vi "BELKIN EAGLE RT Main V1.vi"() -> ()   [LabVIEW 2015]
uses:
  Stream/Controls/RT Status Refs.ctl
  <vilib>/userdefined/High Color/IMAQdx.ctl
  Stream/Controls/RT Streamer Queue element.ctl
  Stream/Controls/RT Streamer State.ctl
  Stream/LP Globals.vi
panel:
  out "Timings":u32[](array[numeric])
  in  "CamSession":T1="cam0"
  in  "AutoBalance":bool
  in  "SetParams":bool
  in  "StatusRefs":T2
  out "output cluster":T3
  in  "AlgoRate":u8=10
  out "FrameRate":dbl
  out "Image Dst Out":T4(plugin-control)
  out "MaxY":u32
  out "MaxX":u32
  out "MaxB":u32
  out "MaxA":u32
  out "HorCenter":u16
  out "VerCenter":u32
  out "Algo Time":u32
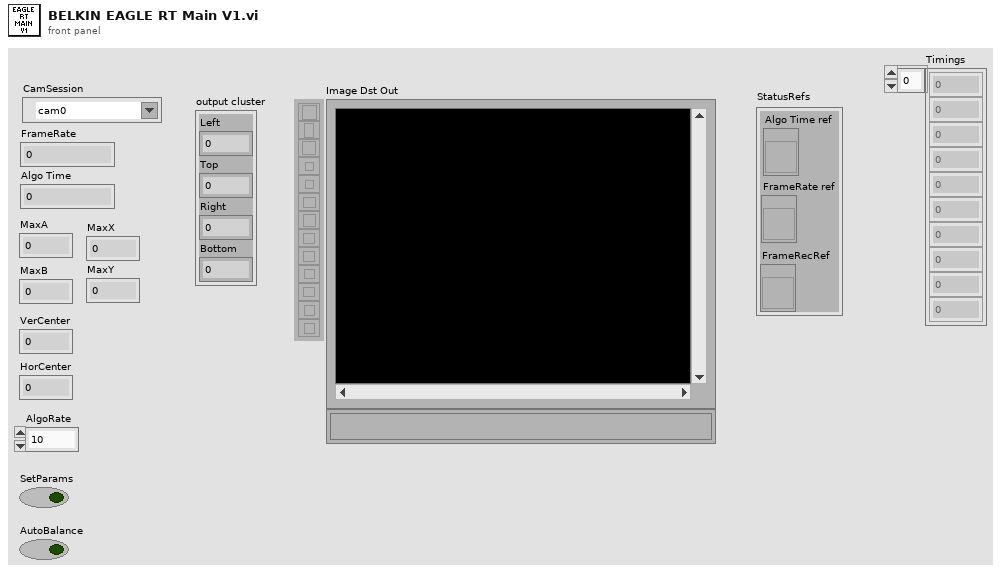
[diagram p1: front panel]
types:
  T1 = typedef "IMAQdx.ctl" = refnum<k21>
  T2 = typedef "RT Status Refs.ctl" = cluster{"Algo Time ref":refnum<vi>, "FrameRate ref":refnum<vi>, "FrameRecRef":refnum<vi>}
  T3 = cluster{"Left":i32, "Top":i32, "Right":i32, "Bottom":i32}
  T4 = typedef "IMAQ Image.ctl" = refnum<image>
  T5 = typedef "RT Streamer Queue element.ctl" = cluster{"CMD":T6, "Data":variant}
  T6 = typedef "RT Streamer State.ctl" = enum16{"Init", "Idle", "Stream", "Listen", "SetRefrashRate", "SendCmdAck", "SendCmdDone", "SendSysState", "StartRecord", "Error"}
  T7 = typedef "Image Type" = u32
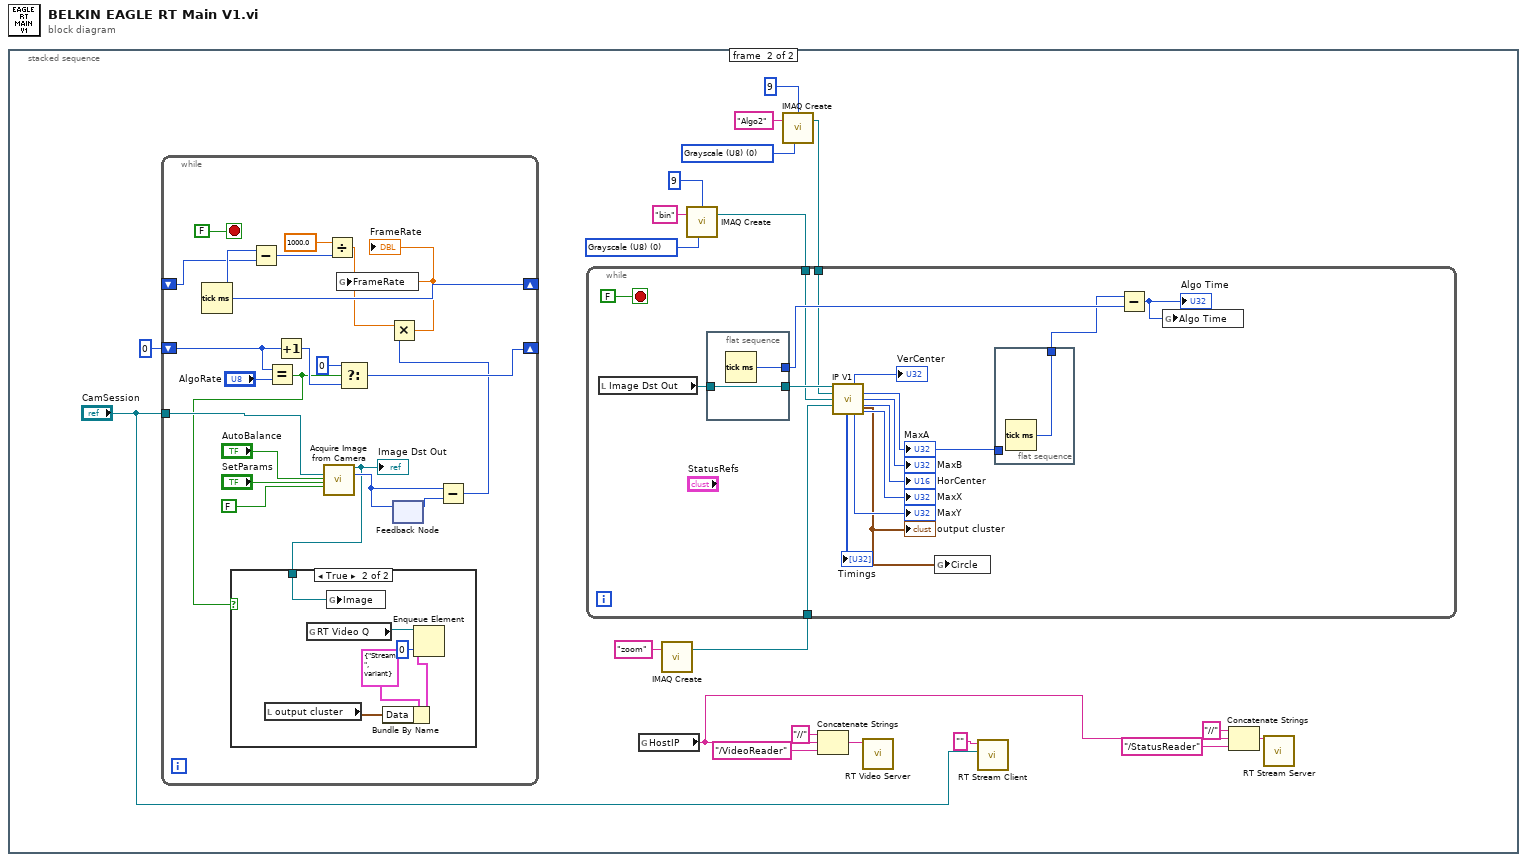
[diagram p0: block diagram]
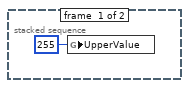
[diagram p2: hidden frame]
diagram:
  n1 = stacked-sequence {
    frame #0 {
      n2 = global write "LP Globals.vi" "UpperValue"(255 ("UpperValue")) -> ()
    }
    frame #1 {
      w8 = T7 0 items=["Grayscale (U8)", "Grayscale (I16)", "Grayscale (SGL)", "Complex (CSG)", "RGB (U32)", "HSL (U32)", "RGB (U64)", "Grayscale (U16)"] ("Image Type")
      w12 = T7 0 items=["Grayscale (U8)", "Grayscale (I16)", "Grayscale (SGL)", "Complex (CSG)", "RGB (U32)", "HSL (U32)", "RGB (U64)", "Grayscale (U16)"] ("Image Type")
      n3 = while {
        shift-right: [w60] -> _
        shift-left: _ -> [w59]
        shift-right: [w55] -> _
        shift-left: u8 0 -> [w57]
        tunnel: "CamSession" -> [w44]
        stop <- FALSE stop-if-true
        n4 = Tick Count (ms)() -> (millisecond timer value=w60:u32)
        n5 = Subtract(x=w60, y=w59) -> (x-y=w58:u32)
        n6 = Equal?(x=w57, y="AlgoRate") -> (x = y?=w43:bool)
        n7 = Increment(x=w57) -> (x+1=w56:u8)
        n8 = call "Acquire Image from Camera.vi"("Session In"=w44, "AutoBalance"="AutoBalance", "Set"="SetParams", "Stop (F)"=FALSE) -> ("Image Out"=w42:T4, "Buffer Number Out"=w48:u32)  [unwired: 20 in, 2 out]
        "Image Dst Out" <- w42
        n9 = case shown="True" w43 {
          tunnel: w42 -> [_ w64]
          frame False {
          }
          frame True {
            n10 = local read "output cluster"() -> (w65:T3)
            n11 = global read "LP Globals.vi" "RT Video Q"() -> (w68:refnum<queue>)
            n12 = global write "LP Globals.vi" "Image"(w64) -> ()
            n13 = Bundle By Name(cluster=T5 {"CMD"=enum."Stream", "Data"=variant} ("element"), "Data"=w65) -> (w66:T5)
            n14 = Enqueue Element(queue=w68, element=w66, timeout in ms (-1)=0) -> ()  [unwired: 1 in, 3 out]
          }
        }
        n15 = Divide(x=1000.0, y=w58) -> (x/y=w49:dbl)
        n16 = Select(t=u8 0, s=w43, f=w56) -> (s? t:f=w55:u8)
        n17 = feedback-in #1(w48) -> ()
        n18 = feedback #1() -> (w47:u32)  [unwired: 1 in]
        n19 = Subtract(x=w48, y=w47) -> (x-y=w46:u32)
        n20 = Multiply(x=w49, y=w46) -> (x*y=w45:dbl)
        "FrameRate" <- w45
        n21 = global write "LP Globals.vi" "FrameRate"(w45) -> ()
      }
      n22 = global read "LP Globals.vi" "HostIP"() -> (w13:string)
      n23 = call "IMAQ Create"("Image Name"="zoom") -> ("New Image"=w3:T4)  [unwired: 3 in, 2 out]
      n24 = call "IMAQ Create"("Border Size"=9, "Image Name"="bin", "Image Type"=w8) -> ("New Image"=w7:T4)  [unwired: 2 in, 1 out]
      n25 = call "IMAQ Create"("Border Size"=9, "Image Name"="Algo2", "Image Type"=w12) -> ("New Image"=w10:T4)  [unwired: 2 in, 1 out]
      n26 = while {
        tunnel: w10 -> [w29]
        tunnel: w7 -> [w28]
        tunnel: w3 -> [w25]
        stop <- FALSE stop-if-true
        n27 = local read "Image Dst Out"() -> (w23:T4)
        n28 = flat-sequence {
          tunnel: [w41] -> w32
          tunnel: w23 -> [w40]
          tunnel: [w40] -> w30
          frame #0 {
            n29 = Tick Count (ms)() -> (millisecond timer value=w41:u32)
          }
        }
        n30 = call "IP V1.vi"("Image In"=w30, "Image Dst"=w29, "BinImage"=w28, "Zoom Image"=w25) -> ("VerCenter"=→"VerCenter":u32, "MaxA"=w27:u32, "MaxB"=→"MaxB":u32, "HorCenter"=→"HorCenter":u16, "Timings"=→"Timings":u32[], "output cluster"=w22:T3, "MaxY"=→"MaxY":u32, "MaxX"=→"MaxX":u32)  [unwired: 1 in, 3 out]
        "MaxA" <- w27
        "output cluster" <- w22
        n31 = global write "LP Globals.vi" "Circle"(w22) -> ()
        n32 = flat-sequence {
          tunnel: [w39] -> w31
          tunnel: w27 -> [_]
          frame #0 {
            n33 = Tick Count (ms)() -> (millisecond timer value=w39:u32)
          }
        }
        n34 = Subtract(x=w31, y=w32) -> (x-y=w26:u32)
        "Algo Time" <- w26
        n35 = global write "LP Globals.vi" "Algo Time"(w26) -> ()
      }
      n36 = Concatenate Strings("//" ("string"), w13, "/VideoReader" ("reader url")) -> (w18:string)
      n37 = call "RT Video Server.vi"("reader url"=w18) -> ()  [unwired: 11 in]
      n38 = call "RT Stream Client.vi"("CamSession"="CamSession", "Writer url"="") -> ()  [unwired: 10 in]
      n39 = Concatenate Strings("//" ("string"), w13, "/StatusReader" ("reader url")) -> (w15:string)
      n40 = call "RT Stream Server.vi"("reader url"=w15) -> ()  [unwired: 11 in]
    }
  }
